vi "merge_One Shot Rising with Input.vi"   [LabVIEW 2020, in "NI_FunctionBlockMergeVIs.lvlib"]
doc: "Detects a rising edge, a transition from FALSE to TRUE, on the input signal. When a rising edge occurs, <B>output</B> is TRUE for one function block execution. The value of <B>output</B> remains FALSE until a new rising edge occurs."
uses:
  <vilib>/functionblocks/NI_FunctionBlockMergeVIs.lvlib
  <vilib>/functionblocks/FB Core/FB Core.xnode
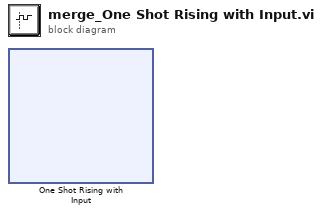
[diagram p0: block diagram]
diagram:
  n1 = xnode "One Shot Rising with Input"() -> ()  [unwired: 2 in, 2 out]
